vi "TPKT - Response Header Mismatch--error.vi"() -> (0 "error out":errorcluster)   [LabVIEW 2014, in "S7NetCom.lvclass"]
doc: "____\nCopyright (c) 2019 Hampel Software Engineering (HSE), released under BSD license. More info can be found on https://dokuwiki.hampel-soft.com/code/hse/s7netcom. Original code published by Marc Christenson, Sisu Devices."
uses:
  S7NetCom.lvclass
panel:
  # "More info on https://dokuwiki.hampel-soft.com/code/hse/s7netcom\n\nCopyright (c) 2019, HAMPEL SOFTWARE ENGINEERING (HSE)\nOriginal code developed by Marc Christenson, Sisu Devices\nAll rights reserved.\n\nRedistribution and use in source and binary forms, with or without\nmodification, are permitted provided that the following conditions are met:\n\n1. Redistributions of source code must retain the above copyright\n   notice, this list of conditions and the following disclaimer.\n\n2. Redistributions in binary form must reproduce the above copyright\n   notice, this list of conditions and the following disclaimer in the\n   documentation and/or other materials provided with the distribution.\n\n3. All advertising materials mentioning features or use of this software\n   must display the following acknowledgement:\n   This product includes software developed by HAMPEL SOFTWARE ENGINEERING.\n\n4. Neither the name of HAMPEL SOFTWARE ENGINEERING nor the\n   names of its contributors may be used to endorse or promote products\n   derived from this software without specific prior written permission.\n\nTHIS SOFTWARE IS PROVIDED BY HAMPEL SOFTWARE ENGINEERING ''AS IS'' AND ANY\nEXPRESS OR IMPLIED WARRANTIES, INCLUDING, BUT NOT LIMITED TO, THE IMPLIED\nWARRANTIES OF MERCHANTABILITY AND FITNESS FOR A PARTICULAR PURPOSE ARE\nDISCLAIMED. IN NO EVENT SHALL HAMPEL SOFTWARE ENGINEERING BE LIABLE FOR ANY\nDIRECT, INDIRECT, INCIDENTAL, SPECIAL, EXEMPLARY, OR CONSEQUENTIAL DAMAGES\n(INCLUDING, BUT NOT LIMITED TO, PROCUREMENT OF SUBSTITUTE GOODS OR SERVICES;\nLOSS OF USE, DATA, OR PROFITS; OR BUSINESS INTERRUPTION) HOWEVER CAUSED AND\nON ANY THEORY OF LIABILITY, WHETHER IN CONTRACT, STRICT LIABILITY, OR TORT\n(INCLUDING NEGLIGENCE OR OTHERWISE) ARISING IN ANY WAY OUT OF THE USE OF THIS\nSOFTWARE, EVEN IF ADVISED OF THE POSSIBILITY OF SUCH DAMAGE."
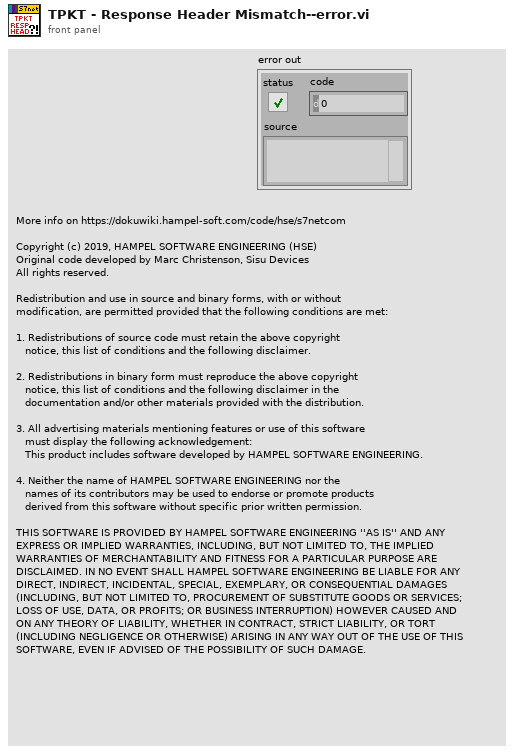
[diagram p1: front panel]
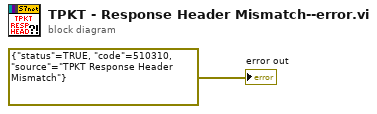
[diagram p0: block diagram]
diagram:
  "error out" <- errorcluster {"status"=TRUE, "code"=510310, "source"="TPKT Response Header Mismatch"} ("error out")
